vi "Soil Monitor Main Program.vi"() -> ()   [LabVIEW 2012]
uses:
  <vilib>/userdefined/High Color/IMAQdx.ctl
  <vilib>/vision/driver/NI_Vision_Acquisition_Software.lvlib
panel:
  out "appended path":path
  out "Image number":i32
  in  "Start Saving Images":bool
  in  "Image Folder Path":path
  in  "Camera time interval (s)":dbl=1.0 min=1.0 max=600.0 step=1.0
  out "Image":T1(plugin-control)
  in  "Camera Name":T2="cam0"
  out "Waveform Chart":dbl(graph)
  out "refnum out":refnum<file>
  in  "Units (0: Gram)":u16(ring) items=["Gram (g)", "Ounce (oz)", "Troy Ounce (oz t)", "Pennyweight (dwt)", "Parts Counting (PC)", "Pound (lb)", "Newton (N)", "Kilogram (kg)", "lb or oz on some models", "Percent (%)"]
  in  "Serial Configuration":T3={"Baud Rate (2400)"=2400, "Flow Control (2: RTS/CTS)"=2, "Parity (0: None)"=0, "Data Bits (7)"=7} {"Data Bits (7)" items=["7"=7, "8"=8]; "Parity (0: None)" items=["None", "Odd", "Even"]; "Flow Control (2: RTS/CTS)" items=["None", "XON/XOFF", "RTS/CTS"]; "Baud Rate (2400)" items=["600"=600, "1200"=1200, "2400"=2400, "4800"=4800, "9600"=9600, "19200"=19200]}
  in  "VISA resource name":refnum<visa-resource-name>="Ohaus_scale"
  out "Stable?":bool
  out "Units":string
  out "Weight Value":dbl format="%.2g"
  out "stop":bool
  in  "Data file path":path
  in  "Start Saving Scale Data":bool
  in  "Quit":bool
  in  "Scale time interval (s)":dbl=1.0 min=1.0 max=600.0 step=1.0
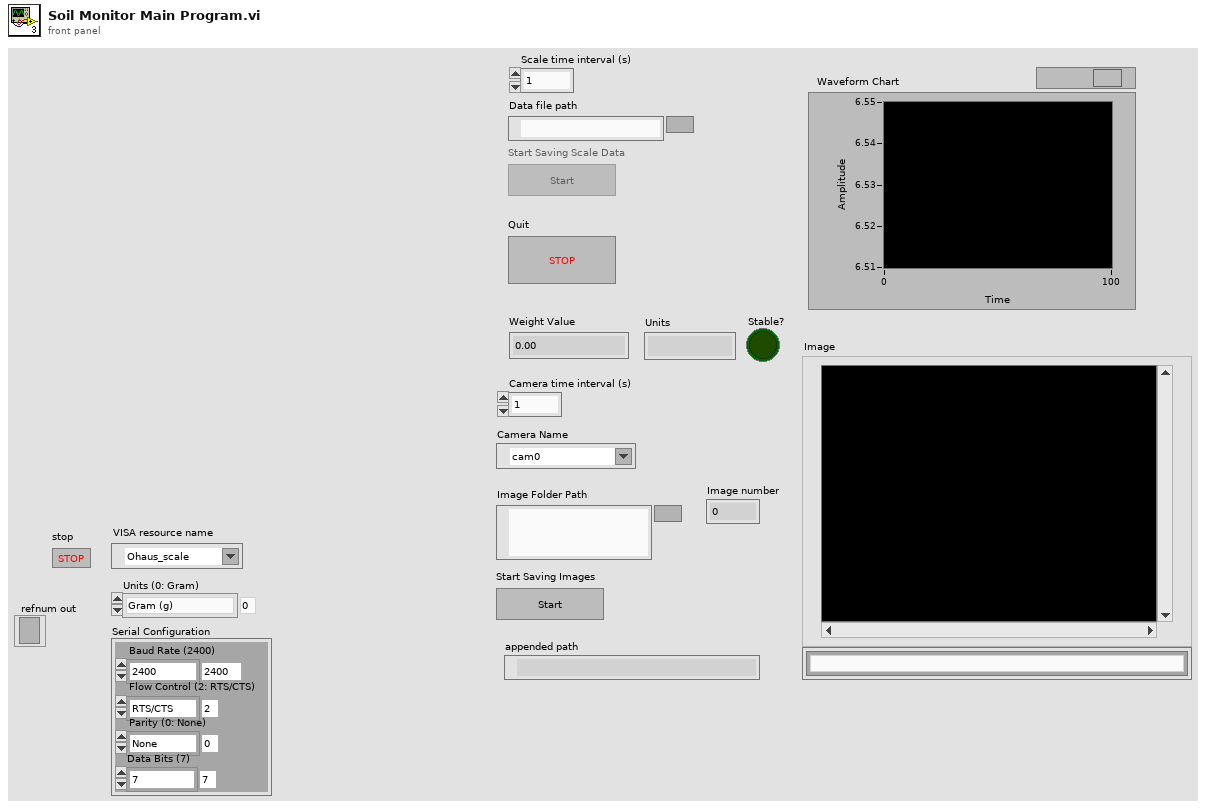
[diagram p1: front panel]
types:
  T1 = typedef "IMAQ Image.ctl" = refnum<image>
  T2 = typedef "IMAQdx.ctl" = refnum<k21>
  T3 = cluster{"Baud Rate (2400)":u32, "Flow Control (2: RTS/CTS)":u16, "Parity (0: None)":u16, "Data Bits (7)":u16}
  T4 = enum16{"open", "replace", "create", "open or create", "replace or create", "replace or create with confirmation"}
  T5 = enum8{"Enabled", "Disabled", "Disabled and Grayed Out"}
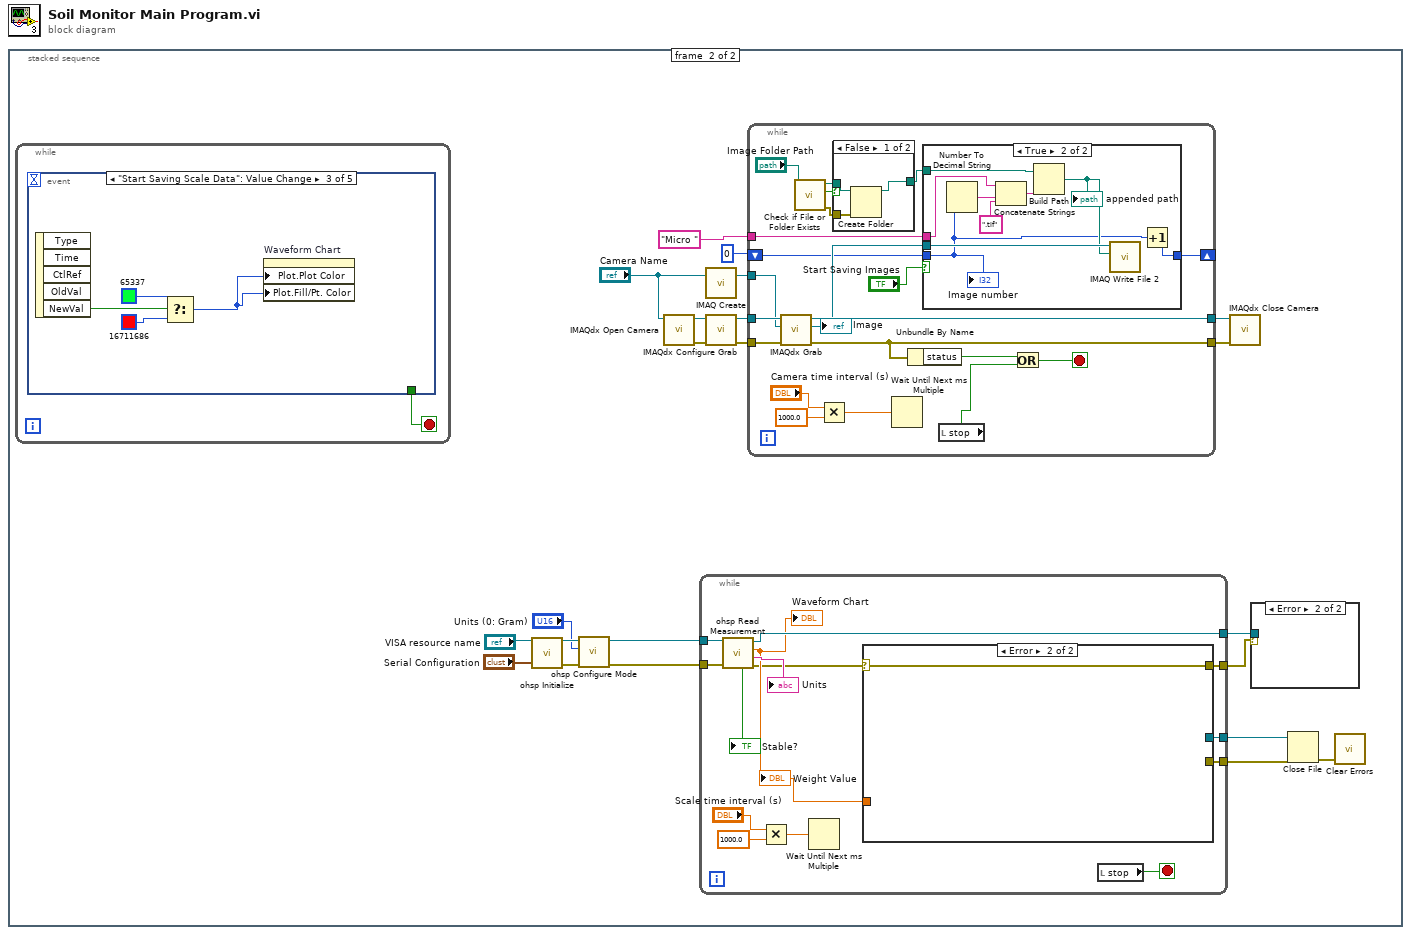
[diagram p0: block diagram]
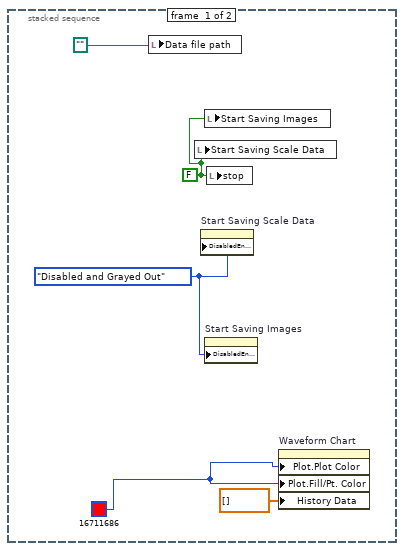
[diagram p2: hidden frame]
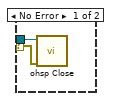
[diagram p3: hidden frame]
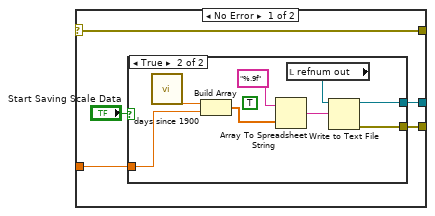
[diagram p6: hidden frame]
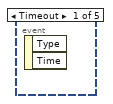
[diagram p8: hidden frame]
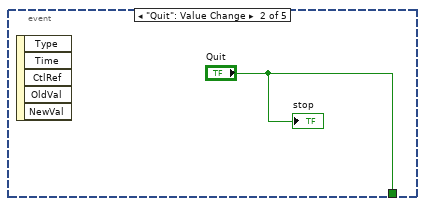
[diagram p9: hidden frame]
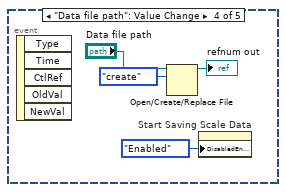
[diagram p10: hidden frame]
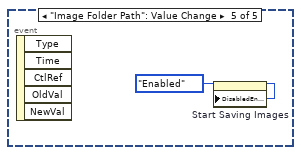
[diagram p11: hidden frame]
diagram:
  n1 = stacked-sequence {
    frame #0 {
      w2 = u32 16711686
      w4 = T5."Disabled and Grayed Out" ("Disabled")
      w3 = FALSE ("stop")
      n2 = local write "Data file path"(path "") -> ()
      n3 = local write "Start Saving Scale Data"(w3) -> ()
      n4 = property on="Start Saving Scale Data" class="Bool (strict)"("DisabledEnum"=w4) -> ()  [unwired: 2 in, 2 out]
      n5 = local write "Start Saving Images"(w3) -> ()
      n6 = property on="Start Saving Images" class="Bool (strict)"("DisabledEnum"=w4) -> ()  [unwired: 2 in, 2 out]
      n7 = local write "stop"(w3) -> ()
      n8 = property on="Waveform Chart" class="WFChart (strict)"("Plot.Plot Color"=w2, "Plot.Fill/Pt. Color"=w2, "History Data"=dbl[] []) -> ()  [unwired: 2 in, 2 out]
    }
    frame #1 {
      n9 = while {
        stop <- w93 stop-if-true
        n10 = event shown="[2] \"Start Saving Scale Data\": Value Change" {
          selector: _ -> [_ _ _ _ _]
          dyn-events: _ -> [_ _ _ _ _]
          timeout: _ -> [_ _ _ _ _]
          tunnel: [_ "Quit" _ _ _] -> w93
          event Timeout {
            n11 = event-data() -> ()  [unwired: 1 in, 2 out]
          }
          event "Quit": Value Change {
            n12 = event-data() -> ()  [unwired: 1 in, 5 out]
            "stop" <- "Quit"
          }
          event "Start Saving Scale Data": Value Change {
            n13 = event-data() -> ("NewVal"=w98:bool)  [unwired: 1 in, 4 out]
            n14 = Select(t=u32 65337, s=w98, f=u32 16711686) -> (s? t:f=w95:u32)
            n15 = property on="Waveform Chart" class="WFChart (strict)"("Plot.Plot Color"=w95, "Plot.Fill/Pt. Color"=w95) -> ()  [unwired: 2 in, 2 out]
          }
          event "Data file path": Value Change {
            n16 = event-data() -> ()  [unwired: 1 in, 5 out]
            n17 = Open/Create/Replace File(file path (use dialog)="Data file path", operation (0:open)=T4."create") -> (refnum out=→"refnum out":refnum<file>)  [unwired: 4 in, 2 out]
            n18 = property on="Start Saving Scale Data" class="Bool (strict)"("DisabledEnum"=T5."Enabled" ("Disabled")) -> ()  [unwired: 2 in, 2 out]
          }
          event "Image Folder Path": Value Change {
            n19 = event-data() -> ()  [unwired: 1 in, 5 out]
            n20 = property on="Start Saving Images" class="Bool (strict)"("DisabledEnum"=T5."Enabled" ("Disabled")) -> ()  [unwired: 2 in, 2 out]
          }
        }
      }
      n21 = call <instrlib>:"ohsp Initialize.vi"("VISA resource name"="VISA resource name", "Serial Configuration"="Serial Configuration") -> ("VISA resource name out"=w26:refnum<visa-resource-name>, "error out"=w27:errorcluster)  [unwired: 12 in]
      n22 = call <instrlib>:"ohsp Configure Mode.vi"("error in (no error)"=w27, "Units (0: Gram)"="Units (0: Gram)", "VISA resource name"=w26) -> ("error out"=w21:errorcluster, "VISA resource name out"=w22:refnum<visa-resource-name>)  [unwired: 7 in]
      n23 = call <vilib>:"IMAQdx Open Camera.vi"("Session In"="Camera Name") -> ("error out"=w14:errorcluster, "Session Out"=w15:T2)  [unwired: 2 in, 7 out]
      n24 = while {
        tunnel: w22 -> [w74]
        tunnel: w21 -> [w73]
        tunnel: [w70] -> w20
        tunnel: [w65] -> w6
        tunnel: [w69] -> w19
        tunnel: [w68] -> w18
        stop <- w75 stop-if-true
        n25 = call <instrlib>:"ohsp Read Measurement.vi"("error in (no error)"=w73, "VISA resource name"=w74) -> ("error out"=w66:errorcluster, "Units"=→"Units":string, "Weight Value"=w67:dbl, "VISA resource name out"=w70:refnum<visa-resource-name>, "Stable?"=→"Stable?":bool)  [unwired: 5 in]
        "Weight Value" <- w67
        "Waveform Chart" <- w67
        n26 = Multiply(x="Scale time interval (s)", y=1000.0) -> (x*y=w76:dbl)
        n27 = Wait Until Next ms Multiple(millisecond multiple=w76) -> ()  [unwired: 1 out]
        n28 = case shown="Error" w66 {
          selector: w66 -> [w79 w92]
          tunnel: [w83 _] -> w69
          tunnel: [w82 _] -> w68
          tunnel: w67 -> [w80 _]
          tunnel: [w79 w92] -> w65
          frame No Error {
            n29 = case shown="True" "Start Saving Scale Data" {
              tunnel: w80 -> [_ w90]
              tunnel: [_ w86] -> w83
              tunnel: [_ w85] -> w82
              frame False {
              }
              frame True {
                (unwired) TRUE ("append to file? (new file:F)")
                n30 = call "days since 1900.vi"() -> ("fractional days"=w91:ext)  [unwired: 11 in]
                n31 = Build Array(w91, w90) -> (w89:ext[])
                n32 = Array To Spreadsheet String(array=w89, 3:"%.9f" ("format string")) -> (spreadsheet string=w88:string)  [unwired: 1 in]
                n33 = local read "refnum out"() -> (w87:refnum<file>)
                n34 = Write to Text File(file (use dialog)=w87, text=w88) -> (refnum out=w86:refnum<file>, error out=w85:errorcluster)  [unwired: 2 in, 1 out]
              }
            }
          }
          frame Error {
          }
        }
        n35 = local read "stop"() -> (w75:bool)
      }
      n36 = call "IMAQ Create"("Image Name"="Camera Name") -> ("New Image"=w9:T1)  [unwired: 3 in, 2 out]
      n37 = call <vilib>:"IMAQdx Configure Grab.vi"("error in"=w14, "Session In"=w15) -> ("error out"=w11:errorcluster, "Session Out"=w10:T2)  [unwired: 8 out]
      n38 = while {
        tunnel: [w45] -> w12
        tunnel: w11 -> [w47]
        tunnel: w10 -> [w48]
        tunnel: [w44] -> w13
        tunnel: w9 -> [w46]
        tunnel: "Micro " -> [w35]
        shift-right: [w37] -> _
        shift-left: 0 -> [w36]
        stop <- w50 stop-if-true
        n39 = call <vilib>:"IMAQdx Grab.vi"("error in"=w47, "Image In"=w46, "Session In"=w48) -> ("error out"=w44:errorcluster, "Image Out"=w39:T1, "Session Out"=w45:T2)  [unwired: 1 in, 5 out]
        "Image" <- w39
        n40 = call <vilib>:"Check if File or Folder Exists.vi"("path"="Image Folder Path") -> ("error out"=w33:errorcluster, "file or folder exists?"=w31:bool, "dup path"=w32:path)  [unwired: 8 in]
        n41 = Multiply(x="Camera time interval (s)", y=1000.0) -> (x*y=w43:dbl)
        n42 = case shown="False" w31 {
          tunnel: w33 -> [w53 _]
          tunnel: w32 -> [w52 w54]
          tunnel: [w51 w54] -> w30
          frame False {
            n43 = Create Folder(path (use dialog)=w52, error in=w53) -> (created path=w51:path)  [unwired: 1 in, 2 out]
          }
          frame True {
          }
        }
        n44 = Wait Until Next ms Multiple(millisecond multiple=w43) -> ()  [unwired: 1 out]
        n45 = Unbundle By Name(w44) -> ("status"=w49:bool)
        n46 = case shown="True" "Start Saving Images" {
          tunnel: w39 -> [_ w64]
          tunnel: w30 -> [_ w60]
          tunnel: [w55 w61] -> w37
          tunnel: w36 -> [w55 w57]
          tunnel: w35 -> [_ w58]
          frame False {
          }
          frame True {
            n47 = Number To Decimal String(number=w57) -> (decimal integer string=w63:string)  [unwired: 1 in]
            n48 = Concatenate Strings(w58, w63, ".tif" ("string")) -> (w62:string)
            n49 = Build Path(base path=w60, name or relative path=w62) -> (appended path=w59:path)
            "appended path" <- w59
            n50 = call-poly "IMAQ Write File 2"("File Path"=w59, "Image"=w64) -> ()  [unwired: 8 in, 2 out]
            n51 = Increment(x=w57) -> (x+1=w61:i32)
            "Image number" <- w57
          }
        }
        n52 = local read "stop"() -> (w40:bool)
        n53 = Or(x=w49, y=w40) -> (x .or. y?=w50:bool)
      }
      n54 = call <vilib>:"IMAQdx Close Camera.vi"("error in"=w13, "Session In"=w12) -> ()  [unwired: 10 out]
      n55 = case shown="Error" w6 {
        selector: w6 -> [w28 _]
        tunnel: w20 -> [w29 _]
        frame No Error {
          n56 = call <instrlib>:"ohsp Close.vi"("error in (no error)"=w28, "VISA resource name"=w29) -> ()  [unwired: 8 in, 1 out]
        }
        frame Error {
        }
      }
      n57 = Close File(refnum=w19, error in=w18) -> (error out=w17:errorcluster)  [unwired: 1 out]
      n58 = call <vilib>:"Clear Errors.vi"("error in (no error)"=w17) -> ()  [unwired: 6 in, 1 out]
    }
  }
